vi "Get InitializationVI Path.vi"(8 "error in (no error)":errorcluster, 11 "Project XML Editor in":refnum<class "Project XML Editor.lvclass">) -> (0 "error out":errorcluster, 1 "Found ?":bool, 2 "Path out":string, 3 "Project XML Editor out":refnum<class "Project XML Editor.lvclass">)   [LabVIEW 2018, in ".LVLIBP CD XML Updater.lvlib" / "Project XML Editor.lvclass"]
uses:
  Project XML Editor.lvclass
  <vilib>/xml/Close Reference(Node).vi
  <vilib>/xml/NI_XML.lvlib
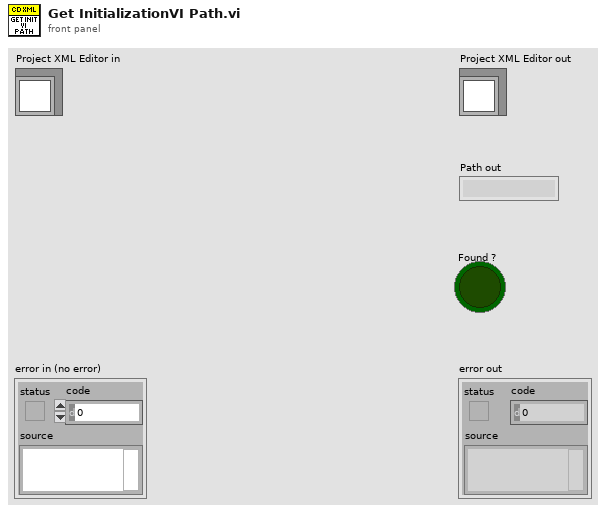
[diagram p1: front panel]
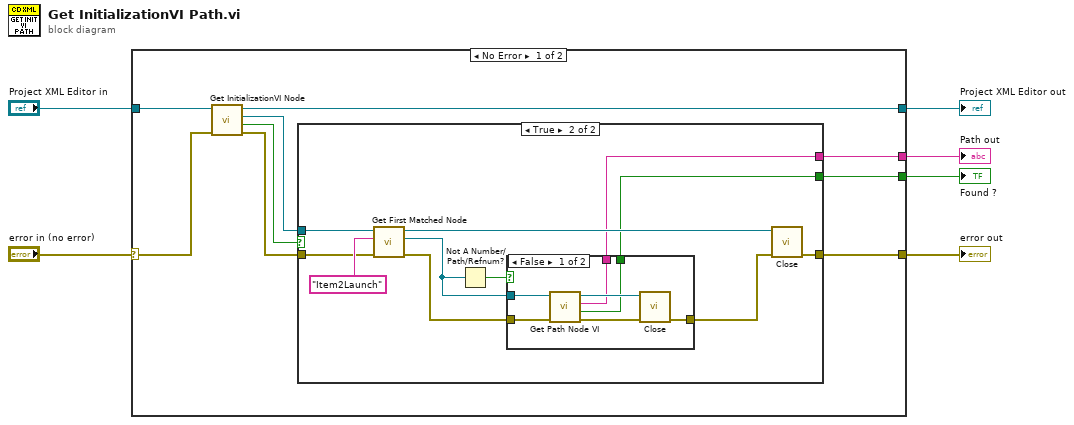
[diagram p0: block diagram]
diagram:
  n1 = case shown="No Error" "error in (no error)" {
    selector: "error in (no error)" -> [w7 w37]
    tunnel: [w13 w37] -> w5
    tunnel: [w11 w36] -> w3
    tunnel: "Project XML Editor in" -> [w12 w36]
    tunnel: [w15 _] -> w2
    tunnel: [w14 _] -> w1
    frame No Error {
      n2 = call "Get InitializationVI Node.vi"("error in (no error)"=w7, "Project XML Editor in"=w12) -> ("error out"=w8:errorcluster, "Found?"=w9:bool, "Node ref out"=w10:refnum<k20>, "Project XML Editor out"=w11:refnum<class "Project XML Editor.lvclass">)  [unwired: 6 in]
      n3 = case shown="True" w9 {
        tunnel: w10 -> [_ w27]
        tunnel: w8 -> [w16 w24]
        tunnel: [_ w21] -> w15
        tunnel: [_ w20] -> w14
        tunnel: [w16 w19] -> w13
        frame False {
        }
        frame True {
          n4 = call <vilib>:"Get First Matched Node.vi"("error in (no error)"=w24, "XPath expression"="Item2Launch", "node in"=w27) -> ("error out"=w23:errorcluster, "node result"=w18:refnum<k20>, "node out"=w25:refnum<k20>)  [unwired: 6 in]
          n5 = Not A Number/Path/Refnum?(number/path/refnum=w18) -> (NaN/Path/Refnum?=w17:bool)
          n6 = case shown="False" w17 {
            tunnel: w23 -> [w32 w35]
            tunnel: [w31 w35] -> w22
            tunnel: [w30 _] -> w21
            tunnel: [w29 _] -> w20
            tunnel: w18 -> [w28 _]
            frame False {
              n7 = call "Get Path Node VI.vi"("error in (no error)"=w32, "Node ref in"=w28) -> ("error out"=w33:errorcluster, "Found ?"=w29:bool, "Path out"=w30:string, "Node ref out"=w34:refnum<k20>)  [unwired: 6 in]
              n8 = call-poly <vilib>:"Close.vi"("error in (no error)"=w33, "node"=w34) -> ("error out"=w31:errorcluster)  [unwired: 7 in]
            }
            frame True {
            }
          }
          n9 = call-poly <vilib>:"Close.vi"("error in (no error)"=w22, "node"=w25) -> ("error out"=w19:errorcluster)  [unwired: 7 in]
        }
      }
    }
    frame Error {
    }
  }
  "error out" <- w5
  "Project XML Editor out" <- w3
  "Path out" <- w2
  "Found ?" <- w1
